vi "Kopie von PH_USB600x_AnalogReader.set timing mode modified.vi"(0 "i ref in":refnum<vi>, 1 "Samples per Channel":i32=1000, 2 "Rate":dbl=10000.0 caption="Rate (Hz)" format="%0.2f", 3 "ms timeout (10000)":i32=10000, 5 "error in (no error)":errorcluster) -> (14 "i ref out":refnum<vi>, 17 "timed out":bool, 19 "error out":errorcluster)   [LabVIEW 2009]
doc: "Sets the timing mode for the scope.\n\nLicense Agreement for this software:\n\nCopyright (C)\nGesellschaft für Schwerionenforschung, GSI\nPlanckstr. 1\n64291 Darmstadt\nGermany\n\nContact: D.Beck@gsi.de \n\nThis program is free software; you can redistribute it and/or modify it under the terms of the GNU General Public License as published by the Free Software Foundation; either version 2 of the license, or (at your option) any later version.\n\nThis program is distributed in the hope that it will be useful, but WITHOUT ANY WARRANTY; without even the implied warranty of MERCHANTABILITY or FITNESS FOR A PARTICULAR PURPOSE. See the GNU General License for more details (http://www.gnu.org).\n\nGesellschaft für Schwerionenforschung, GSI\nPlanckstr. 1, 64291 Darmstadt, Germany\nFor all questions and ideas contact: M.Richter@gsi.de, H.Brand@gsi.de or D.Beck@gsi.de.\nLast update: 17-JUN-2004"
uses:
  PH_USB600x_AnalogReader.lvlib
  <vilib>/DAQmx/configure/timing.llb/DAQmx Timing (Sample Clock).vi
  CSCore/BaseProcess/BaseProcess.lvlib
  lib.lib/DimLVEvent/LVDimInterface/LVDimInterface.lvlib
  CSCore/CSSystem/CSSystemLib/CSSystemLib.lvlib
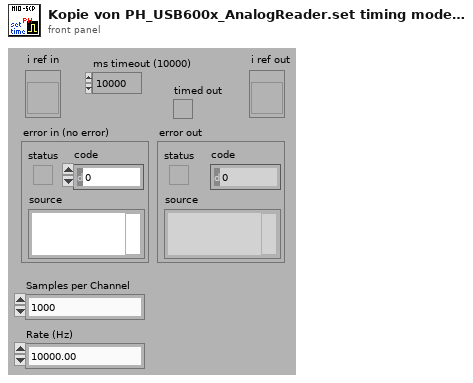
[diagram p1: front panel]
types:
  T1 = typedef "PH_USB600x_AnalogReader.lvlib/PH_USB600x_AnalogReader.i attribute.ctl" = cluster{"GUI Refs":cluster{"Delete":refnum<vi>, "Status":refnum<vi>, "Timeout":refnum<vi>, "Acquire Waveform":refnum<vi>, "Timing":refnum<vi>, "Graph":refnum<vi>, "Prdc Interval":refnum<vi>, "Formula":refnum<vi>}, "Device Settings":cluster{"AIChannel":refnum<k21>, "channelName":string, "Status":T2}, "Timing":T3, "Prdc Interval":dbl, "Lin Scaling":T4, "Data":cluster{"t0":timestamp, dbl}[]}
  T2 = typedef "Status.ctl" = i16
  T3 = typedef "PH_USB600x_AnalogReader.lvlib/PH_USB600x_AnalogReader.Timing.ctl" = cluster{"Samples per Channel":i32, "Rate":dbl}
  T4 = typedef "PH_USB600x_AnalogReader.lvlib/PH_USB600x_AnalogReader.Lin Scaling.ctl" = cluster{"Slope [Unit/V]":dbl, "Offset [Unit]":dbl, "Y-Unit":string, "Y-Label":string}
  T5 = typedef "BaseProcess.lvlib/BaseProcess.i attribute.ctl" = cluster{"EventStatus":string, "EventError":i32, "PresetEvtWatchD":i32, "PresetPdcWatchD":i32, "EventTimeout":i32, "PeriodicInterval":i32, "Interface":string[], "Address":string[], "Special":string[], "PeriodicError":i32, "PeriodicStatus":string, "SuperProc":string, "Descriptors":T6[], "CaseRef":refnum<vi>, "PdcRef":refnum<vi>, "Thread Ref":refnum<vi>, "eventErrorID":i32, "eventStatusID":i32, "periodicErrorID":i32, "periodicStatusID":i32, "pdcCtrID":i32}
  T6 = typedef "BaseProcess.lvlib/BaseProcess.descriptor definition.ctl" = cluster{"selector":string, "descriptor":T7}
  T7 = typedef "BaseProcess.lvlib/BaseProcess.descriptor string definition.ctl" = string
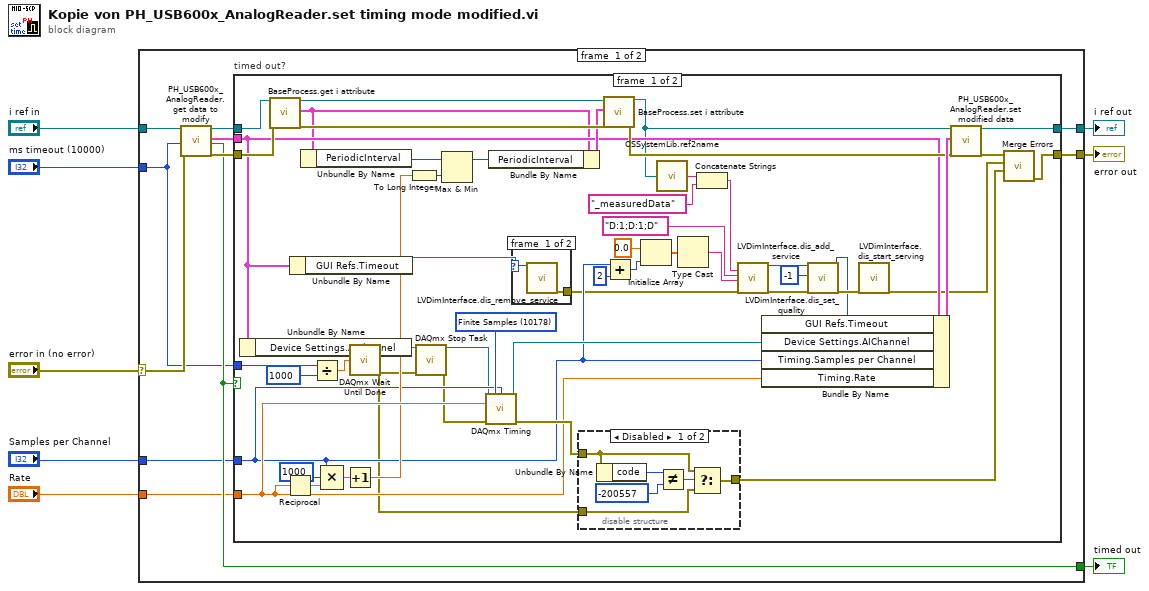
[diagram p0: block diagram]
diagram:
  n1 = case shown="No Error" "error in (no error)" {
    selector: "error in (no error)" -> [w10 w82]
    tunnel: "i ref in" -> [w19 w83]
    tunnel: "ms timeout (10000)" -> [w9 _]
    tunnel: [w17 w83] -> w6
    tunnel: [w15 w82] -> w5
    tunnel: [w14 _] -> w4
    tunnel: "Samples per Channel" -> [w12 _]
    tunnel: "Rate" -> [w11 _]
    frame #0 {
      n2 = call "PH_USB600x_AnalogReader.get data to modify.vi"("i ref in"=w19, "ms timeout (10000)"=w9, "error in (no error)"=w10) -> ("i ref out"=w18:refnum<vi>, "i attribute"=w13:T1, "timed out"=w14:bool, "error out"=w16:errorcluster)  [unwired: 13 in]
      n3 = case "timed out?" shown="False" w14 {
        tunnel: [w53 w81] -> w17
        tunnel: w18 -> [w63 w81]
        tunnel: [w29 w80] -> w15
        tunnel: w16 -> [w62 w80]
        tunnel: w13 -> [w38 _]
        tunnel: w12 -> [w37 _]
        tunnel: w11 -> [w58 _]
        tunnel: w9 -> [w67 _]
        frame #0 {
          w69 = 10178 items=["Finite Samples"=10178, "Continuous Samples"=10123, "Hardware Timed Single Point"=12522] ("sample mode")
          n4 = Unbundle By Name(w38) -> ("Device Settings.AIChannel"=w24:refnum<k21>)
          n5 = call "BaseProcess.get i attribute.vi"("i ref in"=w63, "error in (no error)"=w62) -> ("i ref out"=w61:refnum<vi>, "i attribute"=w28:T5, "error out"=w60:errorcluster)  [unwired: 15 in]
          n6 = Reciprocal(x=w58) -> (1/x=w54:dbl)
          n7 = Unbundle By Name(w38) -> ("GUI Refs.Timeout"=w35:refnum<vi>)
          n8 = Unbundle By Name(w28) -> ("PeriodicInterval"=w27:i32)
          n9 = Divide(x=w67, y=1000) -> (x/y=w68:dbl)
          n10 = Compound Arithmetic op=MULTIPLY(w37, 1000 ("value"), w54) -> (w56:dbl)
          n11 = Increment(x=w56) -> (x+1=w55:dbl)
          n12 = call <vilib>:"DAQmx Wait Until Done.vi"("task/channels in"=w24, "timeout (sec)"=w68) -> ("task out"=w23:refnum<k21>, "error out"=w21:errorcluster)  [unwired: 12 in]
          n13 = To Long Integer(number=w55) -> (32bit integer=w26:i32)
          n14 = call <vilib>:"DAQmx Stop Task.vi"("task/channels in"=w23, "error in"=w21) -> ("task out"=w22:refnum<k21>, "error out"=w20:errorcluster)  [unwired: 12 in]
          n15 = Max & Min(x=w27, y=w26) -> (max(x,y)=w25:i32)  [unwired: 1 out]
          n16 = call-poly <vilib>:"DAQmx Timing.vi"("task/channels in"=w22, "sample mode"=w69, "samples per channel"=w37, "rate"=w58, "error in"=w20) -> ("task out"=w64:refnum<k21>, "error out"=w65:errorcluster)  [unwired: 9 in]
          n17 = Bundle By Name(cluster=w28, "PeriodicInterval"=w25) -> (w59:T5)
          n18 = case shown="Default" w35 {
            selector: w35 -> [w71 _]
            tunnel: [w72 _] -> w36
            frame #0 {
              n19 = call "LVDimInterface.dis_remove_service.vi"("my_serviceID"=w71) -> ("error out"=w72:errorcluster)  [unwired: 18 in]
            }
            frame #1 {
            }
          }
          n20 = disable-structure shown="Disabled" {
            disable-tunnel: w65 -> [w75 w79]
            disable-tunnel: [w74 w79] -> w30
            disable-tunnel: w21 -> [w73 _]
            frame #0 {
              n21 = Unbundle By Name(w75) -> ("code"=w78:i32)
              n22 = Not Equal?(x=w78, y=-200557 ("code")) -> (x != y?=w76:bool)
              n23 = Select(t=w75, s=w76, f=w73) -> (s? t:f=w74:errorcluster)
            }
            frame #1 {
            }
          }
          n24 = call "BaseProcess.set i attribute.vi"("i ref in"=w61, "i attribute"=w59, "error in (no error)"=w60) -> ("i ref out"=w34:refnum<vi>, "error out"=w39:errorcluster)  [unwired: 15 in]
          n25 = Add(x=w37, y=2) -> (x+y=w45:i32)
          n26 = Initialize Array(0.0 ("element"), w45) -> (w46:dbl[])
          n27 = call "CSSystemLib.ref2name.vi"("obj refnum"=w34) -> ("name"=w41:string)
          n28 = Type Cast(x=w46) -> (*(type *) &x=w47:string)  [unwired: 1 in]
          n29 = Concatenate Strings(w41, "_measuredData" ("serviceName")) -> (w48:string)
          n30 = call "LVDimInterface.dis_add_service.vi"("serviceName"=w48, "typeDescriptor"="D:1;D:1;D", "data"=w47, "error in (no error)"=w36) -> ("my_serviceID"=w52:i32, "error out"=w49:errorcluster)  [unwired: 14 in]
          n31 = call "LVDimInterface.dis_set_quality.vi"("my_serviceID"=w52, "quality"=-1, "error in (no error)"=w49) -> ("my_serviceID (out)"=w33:i32, "error out"=w50:errorcluster)  [unwired: 15 in]
          n32 = Bundle By Name(cluster=w38, "GUI Refs.Timeout"=w33, "Device Settings.AIChannel"=w64, "Timing.Samples per Channel"=w37, "Timing.Rate"=w58) -> (w70:T1)
          n33 = call "LVDimInterface.dis_start_serving.vi"("error in (no error)"=w50) -> ("error out"=w31:errorcluster)  [unwired: 17 in, 1 out]
          n34 = call "PH_USB600x_AnalogReader.set modified data.vi"("i ref in"=w34, "i attribute"=w70, "error in (no error)"=w39) -> ("i ref out"=w53:refnum<vi>, "error out"=w32:errorcluster)  [unwired: 15 in]
          n35 = call <vilib>:"Merge Errors.vi"("error in 3 (no error)"=w30, "error in 2 (no error)"=w31, "error in 1 (no error)"=w32) -> ("error out"=w29:errorcluster)  [unwired: 4 in]
        }
        frame #1 {
        }
      }
    }
    frame #1 {
    }
  }
  "error out" <- w5
  "i ref out" <- w6
  "timed out" <- w4
